vi "year_txt.vi"() -> ()   [LabVIEW 2017]
panel:
  in  "year_txt":dbl
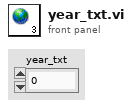
[diagram p1: front panel]
diagram:
